vi "CRYRead from Step to Tree Icon.vi"(3 "Is Refresh?":bool, 4 "StepContentIn":T1(array[cluster]), 5 "StepsRef in":refnum<vi>) -> (2 "StepsRefOut":refnum<vi>)   [LabVIEW 2013]
uses:
  CRYMainGlobal.vi
panel:
  in  "Category":bool
  out "error out":errorcluster
  in  "Index":i32
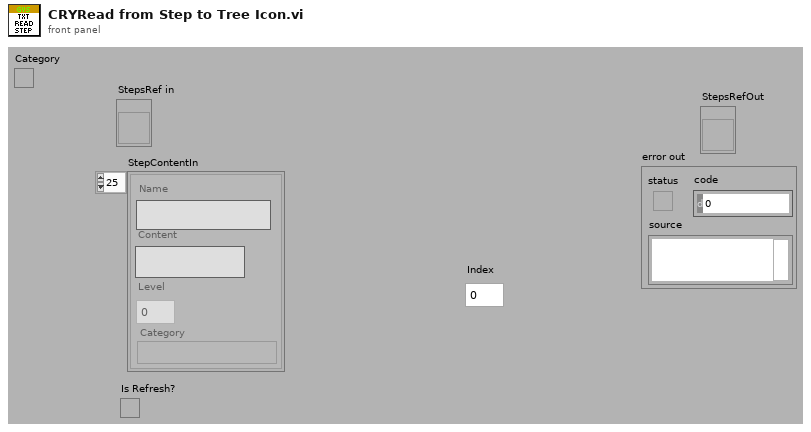
[diagram p1: front panel]
types:
  T1 = cluster{"Content":string, "Name":string, "Level":u32, "Category":string}[]
  T2 = enum32{"English", "Chinese", "Korean", "Japanese", "Russian", "Chinese traditional"}
  T3 = cluster{"Left Cell String":string, "Child Text":string[], "Child Tag":string, "Item Indent":i32, "Child Only?":bool, "Glyph Index":i32}
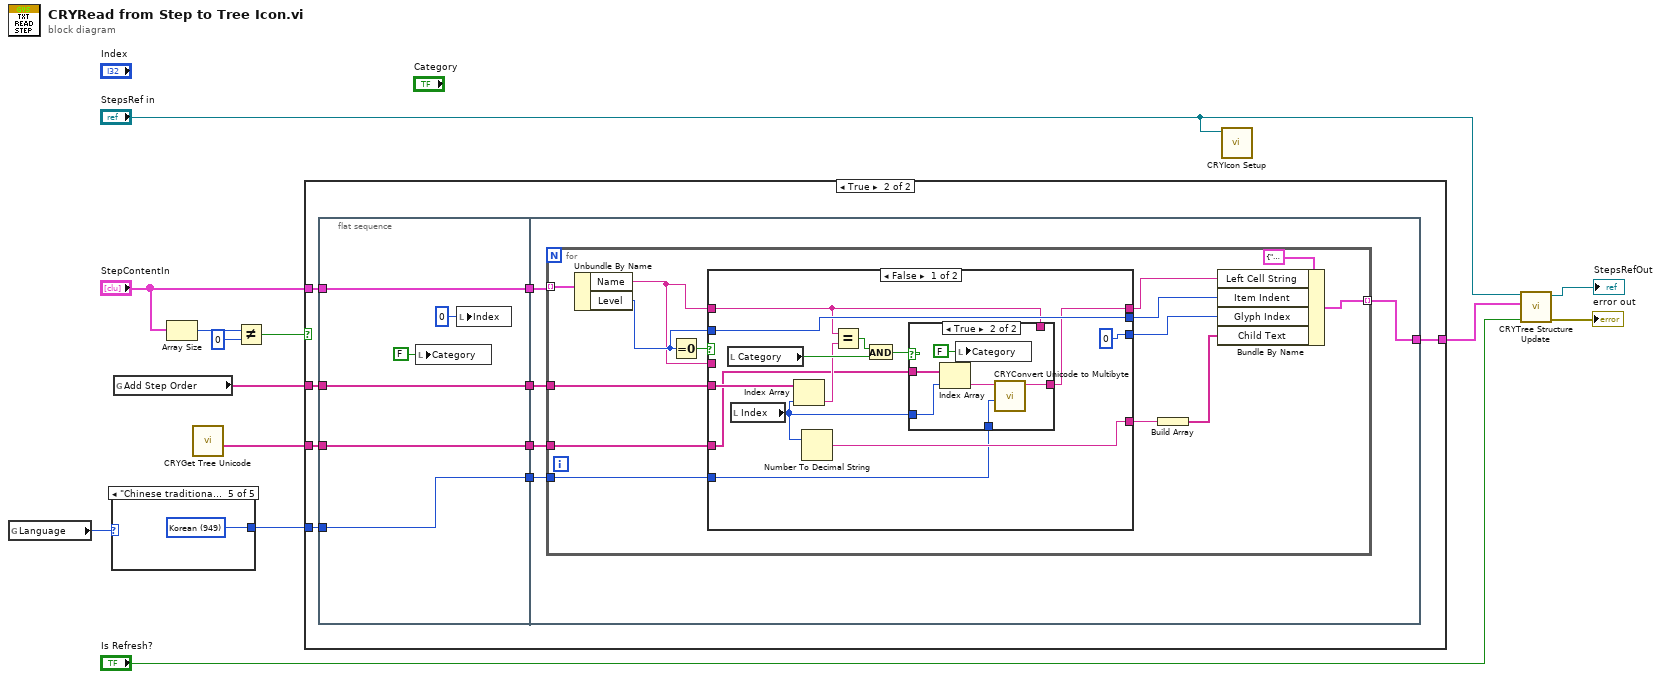
[diagram p0: block diagram]
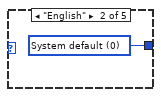
[diagram p3: hidden frame]
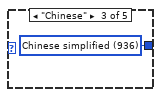
[diagram p4: hidden frame]
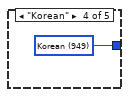
[diagram p5: hidden frame]
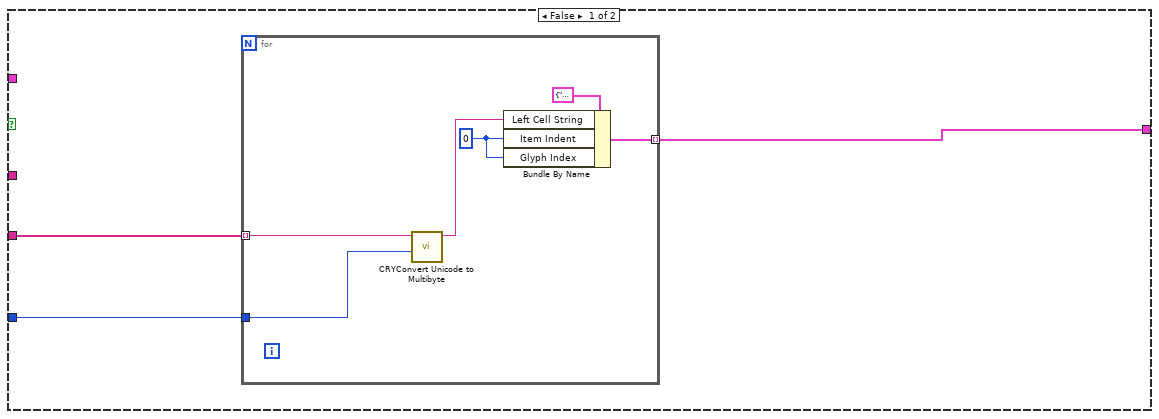
[diagram p6: hidden frame]
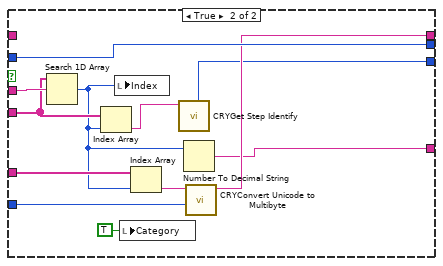
[diagram p8: hidden frame]
diagram:
  n1 = global read "CRYMainGlobal.vi" "Language"() -> (w3:T2)
  n2 = case shown="\"Chinese traditional\"" w3 {
    tunnel: [_ w14 w15 w16 w17] -> w2
    frame Default {
    }
    frame "English" {
      w14 = u32 0 items=["System default"=0, "Latin-1"=1252, "Japanese"=932, "Korean"=949, "Chinese simplified"=936, "Chinese traditional"=950, "Central Europe"=1250, "Cyrillic"=1251, "Greek"=1253, "Turkish"=1254, "Hebrew"=1255, "Arabic"=1256, "Baltic"=1257, "Thai"=874, "Vietnamese"=783, "UTF8"=65001, "UTF-7"=65000] ("Code Page")
    }
    frame "Chinese" {
      w15 = u32 936 items=["System default"=0, "Latin-1"=1252, "Japanese"=932, "Korean"=949, "Chinese simplified"=936, "Chinese traditional"=950, "Central Europe"=1250, "Cyrillic"=1251, "Greek"=1253, "Turkish"=1254, "Hebrew"=1255, "Arabic"=1256, "Baltic"=1257, "Thai"=874, "Vietnamese"=783, "UTF8"=65001, "UTF-7"=65000] ("Code Page")
    }
    frame "Korean" {
      w16 = u32 949 items=["System default"=0, "Latin-1"=1252, "Japanese"=932, "Korean"=949, "Chinese simplified"=936, "Chinese traditional"=950, "Central Europe"=1250, "Cyrillic"=1251, "Greek"=1253, "Turkish"=1254, "Hebrew"=1255, "Arabic"=1256, "Baltic"=1257, "Thai"=874, "Vietnamese"=783, "UTF8"=65001, "UTF-7"=65000] ("Code Page")
    }
    frame "Chinese traditional" {
      w17 = u32 949 items=["System default"=0, "Latin-1"=1252, "Japanese"=932, "Korean"=949, "Chinese simplified"=936, "Chinese traditional"=950, "Central Europe"=1250, "Cyrillic"=1251, "Greek"=1253, "Turkish"=1254, "Hebrew"=1255, "Arabic"=1256, "Baltic"=1257, "Thai"=874, "Vietnamese"=783, "UTF8"=65001, "UTF-7"=65000] ("Code Page")
    }
  }
  n3 = global read "CRYMainGlobal.vi" "Add Step Order"() -> (w4:string[])
  n4 = Array Size(array="StepContentIn") -> (size(s)=w12:i32)
  n5 = call "CRYGet Tree Unicode.vi"() -> ("Unicode Message Sub"=w1:string[])  [unwired: 11 in]
  n6 = Not Equal?(x=w12, y=0) -> (x != y?=w10:bool)
  n7 = case shown="True" w10 {
    tunnel: [w20 w33] -> w8
    tunnel: "StepContentIn" -> [_ w32]
    tunnel: w4 -> [_ w31]
    tunnel: w2 -> [w18 w28]
    tunnel: w1 -> [w19 w27]
    frame False {
      n8 = for {
        tunnel: [w25] -> w20 mode=indexing
        tunnel: w19 -> [w21] mode=indexing
        tunnel: w18 -> [w23]
        w24 = 0 ("Glyph Index")
        n9 = call "CRYConvert Unicode to Multibyte.vi"("Code Page"=w23, "Unicode String"=w21) -> ("Multibyte string"=w22:string)  [unwired: 8 in, 1 out]
        n10 = Bundle By Name(cluster=T3 {"Left Cell String"="", "Child Text"=[], "Child Tag"="", "Item Indent"=0, "Child Only?"=FALSE, "Glyph Index"=0} ("Item"), "Left Cell String"=w22, "Item Indent"=w24, "Glyph Index"=w24) -> (w25:T3)
      }
    }
    frame True {
      n11 = flat-sequence {
        tunnel: w32 -> [w41]
        tunnel: [w39] -> w35
        tunnel: [w41] -> w34
        tunnel: w31 -> [w39]
        tunnel: [w37] -> w30
        tunnel: [w38] -> w29
        tunnel: w28 -> [w38]
        tunnel: w27 -> [w37]
        tunnel: [w44] -> w33
        tunnel: w35 -> [w46]
        tunnel: w34 -> [w45]
        tunnel: w30 -> [w43]
        tunnel: w29 -> [w42]
        frame #0 {
          n12 = local write "Category"(FALSE ("Category")) -> ()
          n13 = local write "Index"(u32 0 ("count")) -> ()
        }
        frame #1 {
          n14 = for {
            tunnel: w45 -> [w55] mode=indexing
            tunnel: [w59] -> w44 mode=indexing
            tunnel: w46 -> [w57]
            tunnel: w43 -> [w50]
            tunnel: w42 -> [w49]
            n15 = Unbundle By Name(w55) -> ("Name"=w53:string, "Level"=w54:u32)
            n16 = Equal To 0?(x=w54) -> (x = 0?=w58:bool)
            n17 = case shown="False" w58 {
              tunnel: w53 -> [_ w92]
              tunnel: [0 ("Symbol Index") w82] -> w56
              tunnel: w57 -> [w69 w84]
              tunnel: w54 -> [w73 w91]
              tunnel: w53 -> [w64 _]
              tunnel: [w63 w88] -> w52
              tunnel: [w73 w91] -> w51
              tunnel: w50 -> [w65 w90]
              tunnel: w49 -> [w61 w87]
              tunnel: [w72 w86] -> w48
              frame False {
                n18 = local read "Category"() -> (w70:bool)
                n19 = local read "Index"() -> (w62:i32)
                n20 = Index Array(array=w69, index=w62) -> (element=w68:string)
                n21 = Number To Decimal String(number=w62) -> (decimal integer string=w72:string)  [unwired: 1 in]
                n22 = Equal?(x=w64, y=w68) -> (x = y?=w67:bool)
                n23 = And(x=w67, y=w70) -> (x .and. y?=w66:bool)
                n24 = case shown="True" w66 {
                  tunnel: w65 -> [_ w79]
                  tunnel: [w74 w78] -> w63
                  tunnel: w64 -> [w74 _]
                  tunnel: w62 -> [_ w76]
                  tunnel: w61 -> [_ w75]
                  frame False {
                  }
                  frame True {
                    n25 = Index Array(array=w79, index=w76) -> (element=w80:string)
                    n26 = local write "Category"(FALSE ("Category")) -> ()
                    n27 = call "CRYConvert Unicode to Multibyte.vi"("Code Page"=w75, "Unicode String"=w80) -> ("Multibyte string"=w78:string)  [unwired: 8 in, 1 out]
                  }
                }
              }
              frame True {
                n28 = Search 1D Array(1D array=w84, element=w92) -> (index of element=w83:i32)  [unwired: 1 out]
                n29 = Index Array(array=w84, index=w83) -> (element=w85:string)
                n30 = local write "Index"(w83) -> ()
                n31 = local write "Category"(TRUE ("Category")) -> ()
                n32 = Index Array(array=w90, index=w83) -> (element=w89:string)
                n33 = call "CRYGet Step Identify.vi"("Category Name In"=w85) -> ("Symbol Index"=w82:i32)  [unwired: 3 in, 7 out]
                n34 = Number To Decimal String(number=w83) -> (decimal integer string=w86:string)  [unwired: 1 in]
                n35 = call "CRYConvert Unicode to Multibyte.vi"("Code Page"=w87, "Unicode String"=w89) -> ("Multibyte string"=w88:string)  [unwired: 8 in, 1 out]
              }
            }
            n36 = Build Array(w48) -> (w47:string[])
            n37 = Bundle By Name(cluster=T3 {"Left Cell String"="", "Child Text"=[], "Child Tag"="", "Item Indent"=0, "Child Only?"=FALSE, "Glyph Index"=0} ("Item"), "Left Cell String"=w52, "Item Indent"=w51, "Glyph Index"=w56, "Child Text"=w47) -> (w59:T3)
          }
        }
      }
    }
  }
  n38 = call "CRYIcon Setup.vi"("TS Tree In"="StepsRef in") -> ()  [unwired: 1 in, 8 out]
  n39 = call "CRYTree Structure Update.vi"("Is Refresh?"="Is Refresh?", "Add Items"=w8, "StepsRef in"="StepsRef in") -> ("error out"=→"error out":errorcluster, "StepsRefOut"=→"StepsRefOut":refnum<vi>)  [unwired: 7 in]
